vi "单精度浮点拆分.vi"(7 "输入":sgl) -> (0 "低字节":u8 format="0x%x", 2 "次低":u8 format="0x%x", 3 "次高":u8 format="0x%x", 4 "小端数组":i32[](array[numeric]), 5 "高字节":u8 format="0x%x")   [LabVIEW 2017]
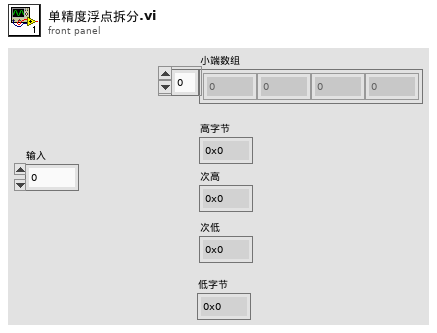
[diagram p1: front panel]
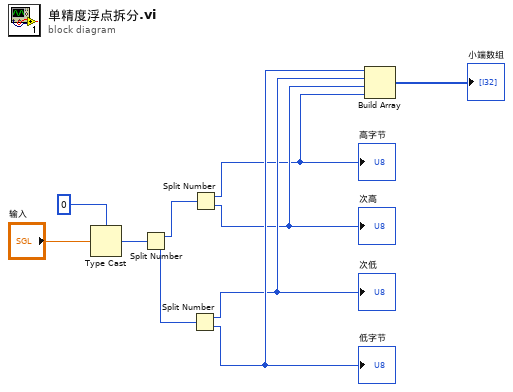
[diagram p0: block diagram]
diagram:
  n1 = Type Cast(type=0, x="输入") -> (*(type *) &x=w8:i32)
  n2 = Split Number(x=w8) -> (hi(x)=w7:u16, lo(x)=w6:u16)
  n3 = Split Number(x=w6) -> (hi(x)=w4:u8, lo(x)=w5:u8)
  "次低" <- w4
  "低字节" <- w5
  n4 = Split Number(x=w7) -> (hi(x)=w2:u8, lo(x)=w3:u8)
  "高字节" <- w2
  "次高" <- w3
  n5 = Build Array(w5, w4, w3, w2) -> (→"小端数组":u8[])
